vi "Restart CCU721 USB Port.vi"(8 "error in (no error)":errorcluster, 10 "Restart?":bool=TRUE, 11 "Device Hardware ID":string="*VID_0483*PID_5740*") -> (0 "error out":errorcluster, 3 "Command Output":string)   [LabVIEW 2011]
doc: "This VI can restart a usb device or disconnect first then scan for new device."
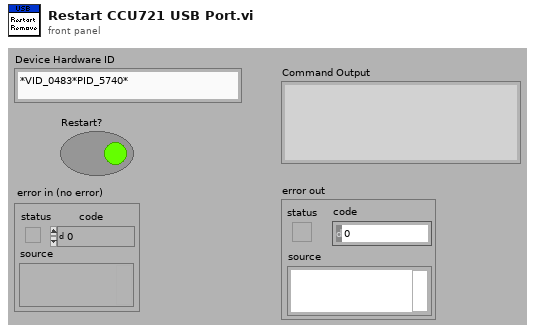
[diagram p1: front panel]
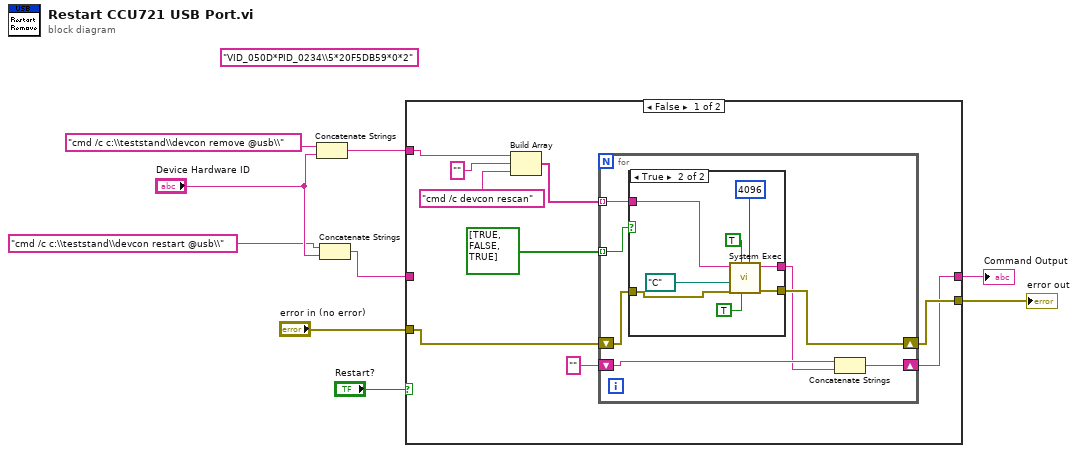
[diagram p0: block diagram]
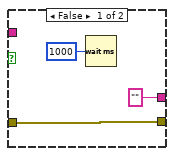
[diagram p2: hidden frame]
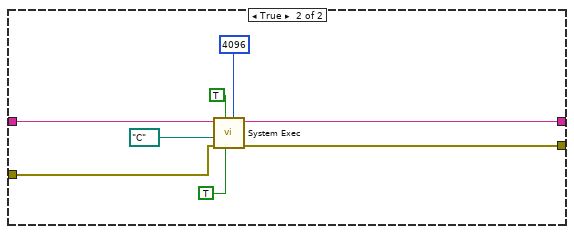
[diagram p3: hidden frame]
diagram:
  (unwired) "VID_050D*PID_0234\\5*20F5DB59*0*2" ("command line")
  n1 = Concatenate Strings("cmd /c c:\\teststand\\devcon remove @usb\\" ("command line"), "Device Hardware ID") -> (w7:string)
  n2 = Concatenate Strings("cmd /c c:\\teststand\\devcon restart @usb\\" ("command line"), "Device Hardware ID") -> (w4:string)
  n3 = case shown="False" "Restart?" {
    tunnel: w7 -> [w18 _]
    tunnel: w4 -> [_ w41]
    tunnel: [w11 w40] -> w1
    tunnel: "error in (no error)" -> [w15 w39]
    tunnel: [w10 w38] -> w2
    frame False {
      n4 = Build Array(w18, "", "cmd /c devcon rescan" ("command line")) -> (w14:string[])
      n5 = for {
        shift-right: [w25] -> w11
        shift-left: w15 -> [w24]
        tunnel: w14 -> [w23] mode=indexing
        tunnel: bool[] [TRUE, FALSE, TRUE] -> [w22] mode=indexing
        shift-right: [w19] -> w10
        shift-left: "" ("standard output") -> [w21]
        n6 = case shown="True" w22 {
          tunnel: ["" ("standard output") w35] -> w20
          tunnel: [w28 w34] -> w25
          tunnel: w24 -> [w28 w31]
          tunnel: w23 -> [_ w30]
          frame False {
            n7 = Wait (ms)(milliseconds to wait=u32 1000) -> ()  [unwired: 1 out]
          }
          frame True {
            n8 = call <vilib>:"System Exec.vi"("expected output size  (4096)"=u32 4096, "run minimized? (F)"=TRUE, "wait until completion? (T)"=TRUE, "error in (no error)"=w31, "working directory"=path "C:/", "command line"=w30) -> ("error out"=w34:errorcluster, "standard output"=w35:string)  [unwired: 2 in, 2 out]
          }
        }
        n9 = Concatenate Strings(w21, w20) -> (w19:string)
      }
    }
    frame True {
      n10 = call <vilib>:"System Exec.vi"("expected output size  (4096)"=u32 4096, "run minimized? (F)"=TRUE, "wait until completion? (T)"=TRUE, "error in (no error)"=w39, "working directory"=path "C:/", "command line"=w41) -> ("error out"=w40:errorcluster, "standard output"=w38:string)  [unwired: 2 in, 2 out]
    }
  }
  "Command Output" <- w2
  "error out" <- w1
